vi "_CSMObj-Update Remaing States.vi"(8 "Error In":errorcluster caption="error in (no error)", 9 "Remaing JKISM Queue":string, 10 "Current State":string, 11 "CSMQ In":T1={"info"={"Module Name"="", "Requested Name"="", "Group Name"="", "Mode"=enum."Stand Alone", "Allowed Messages"=[]}, "Refs"={"WatchDogQ"=refnum, "CSMDataDVR"=refnum, "Queue"={"HPriorityQ"=refnum, "LowPriorityQ"=refnum}, "GroupDataDVR"=refnum, "TagMap"=refnum, "ExitEvent"=refnum, "NewStateEvent"=refnum, "StatusEvent"=refnum, "InterruptEvent"=refnum}}) -> (0 "error out":errorcluster, 1 "Remaing JKISM Queue(dup)":string, 2 "Current State(dup)":string, 3 "CSMQ Out":T1={"info"={"Module Name"="", "Requested Name"="", "Group Name"="", "Mode"=enum."Stand Alone", "Allowed Messages"=[]}, "Refs"={"WatchDogQ"=refnum, "CSMDataDVR"=refnum, "Queue"={"HPriorityQ"=refnum, "LowPriorityQ"=refnum}, "GroupDataDVR"=refnum, "TagMap"=refnum, "ExitEvent"=refnum, "NewStateEvent"=refnum, "StatusEvent"=refnum, "InterruptEvent"=refnum}})   [LabVIEW 2017, in "Communicable State Machine.lvlib"]
uses:
  Communicable State Machine.lvlib
  _CSMObj.ctl
  _CSMObj-Info.ctl
  Typedef/_CSM_MODE.ctl
  _CSMObj-Refs.ctl
  _CSMObj-Data.ctl
  Typedef/_CSM_MSG_TYPE.ctl
  Priority Queue/Priority Queue.ctl
  Typedef/_Cross CSM State Data.ctl
  Typedef/_Cross CSM State Response.ctl
  Typedef/_CSM_Response Source Message.ctl
  Priority Queue/def-Data(LowPRI-Q).ctl
  _CSMObj-ModeData.ctl
  Typedef/_CSM Status Change Event Data.ctl
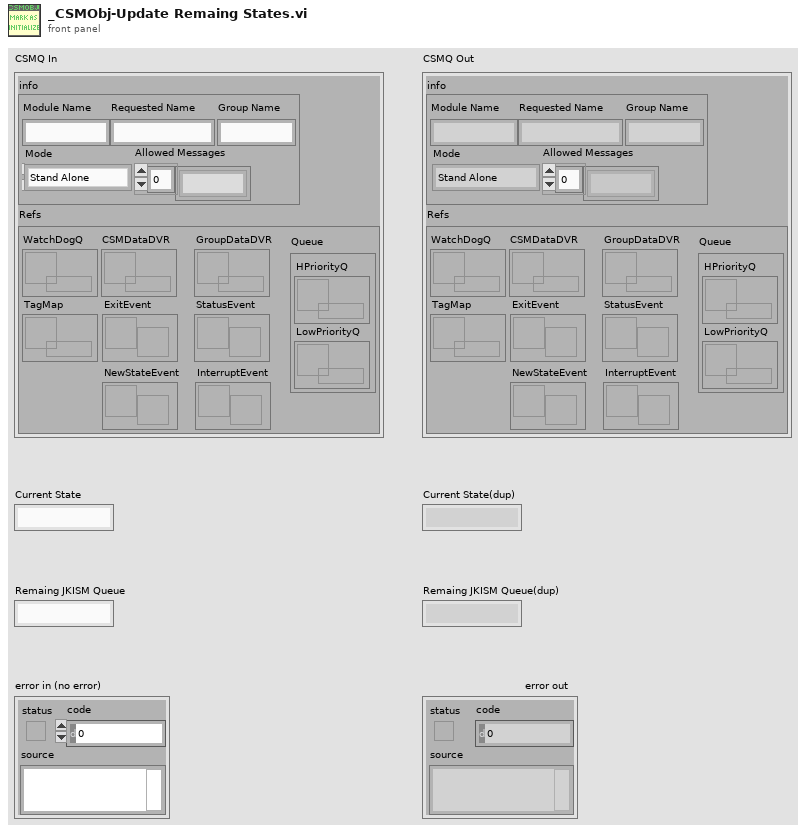
[diagram p1: front panel]
types:
  T1 = typedef "Communicable State Machine.lvlib/_CSMObj.ctl" = cluster{"info":T2, "Refs":T4}
  T2 = typedef "Communicable State Machine.lvlib/_CSMObj-Info.ctl" = cluster{"Module Name":string, "Requested Name":string, "Group Name":string, "Mode":T3, "Allowed Messages":string[]}
  T3 = typedef "Communicable State Machine.lvlib/_CSM_MODE.ctl" = enum16{"Not Exist", "Stand Alone", "CSM", "Worker", "Worker Agent", "Chain Node", "Chain"}
  T4 = typedef "Communicable State Machine.lvlib/_CSMObj-Refs.ctl" = cluster{"WatchDogQ":refnum<queue>, "CSMDataDVR":refnum<data-value>, "Queue":T5, "GroupDataDVR":refnum<data-value>, "TagMap":refnum<data-value>, "ExitEvent":refnum<user-event>, "NewStateEvent":refnum<user-event>, "StatusEvent":refnum<user-event>, "InterruptEvent":refnum<user-event>}
  T5 = typedef "Communicable State Machine.lvlib/Priority Queue.ctl" = cluster{"HPriorityQ":refnum<queue>, "LowPriorityQ":refnum<queue>}
  T6 = typedef "Communicable State Machine.lvlib/_CSMObj-Data.ctl" = cluster{"RemoteMessge?":bool, "error":errorcluster, "Return State":string, "Initialized":enum16{"Initializing", "Ready", "Exiting"}, "InternalRegistryRules":string[], "Return Msg Type":T7, "Current State":string, "Remaing JKISM Queue":string}
  T7 = typedef "Communicable State Machine.lvlib/_CSM_MSG_TYPE.ctl" = enum16{"Sync Message(-@)", "Async Message(->)", "Async without Response(->|)", "Async Response", "Broadcast(-><all>)", "Broadcast(-><status>)", "Broadcast(-><interrupt>)", "Append to JKISM States", "Append to JKISM States(High Priority)", "Broadcast(-><state>)", "<None>"}
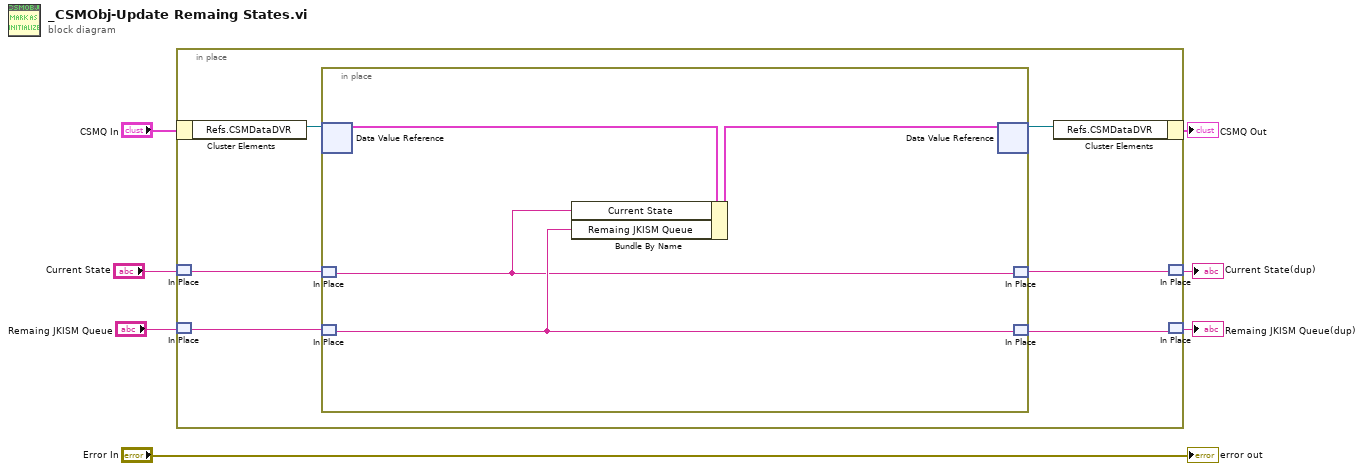
[diagram p0: block diagram]
diagram:
  n1 = in-place "In Place Element Structure" {
    n2 = in-place-cluster #1("CSMQ In") -> ("Refs.CSMDataDVR"=w13:refnum<data-value>)
    n3 = in-place-match #2("Current State") -> (w9:string)
    n4 = in-place-match #3("Remaing JKISM Queue") -> (w11:string)
    n5 = in-place {
      n6 = in-place-dvr #4(w13) -> (w17:T6)  [unwired: 1 out]
      n7 = in-place-match #5(w9) -> (w14:string)
      n8 = in-place-match #6(w11) -> (w15:string)
      n9 = Bundle By Name(cluster=w17, "Current State"=w14, "Remaing JKISM Queue"=w15) -> (w16:T6)
      n10 = in-place-dvr #4(w16) -> (w12:refnum<data-value>)  [unwired: 1 out]
      n11 = in-place-match #5(w14) -> (w8:string)
      n12 = in-place-match #6(w15) -> (w10:string)
    }
    n13 = in-place-cluster #1("Refs.CSMDataDVR"=w12) -> (→"CSMQ Out":T1)
    n14 = in-place-match #2(w8) -> (→"Current State(dup)":string)
    n15 = in-place-match #3(w10) -> (→"Remaing JKISM Queue(dup)":string)
  }
  "error out" <- "Error In"
